vi "WorkTable Sandbox.vi"() -> ()   [LabVIEW 2011]
uses:
  Vec3d Class/Vec3d Class.lvclass
  WorkTable Class.lvclass
panel:
  out "Syringe":T1
  out "Tool Rack":T2
  in  "Config Folder":path=path "C:/Users/husker/Desktop/gantry/Config"
  out "Weights":T3
  out "Stamps":T4
  out "Manifold":T5
  out "BBM":T6
  out "Glue Reservoir":T7
  out "error out":errorcluster
  out "HDI":T8
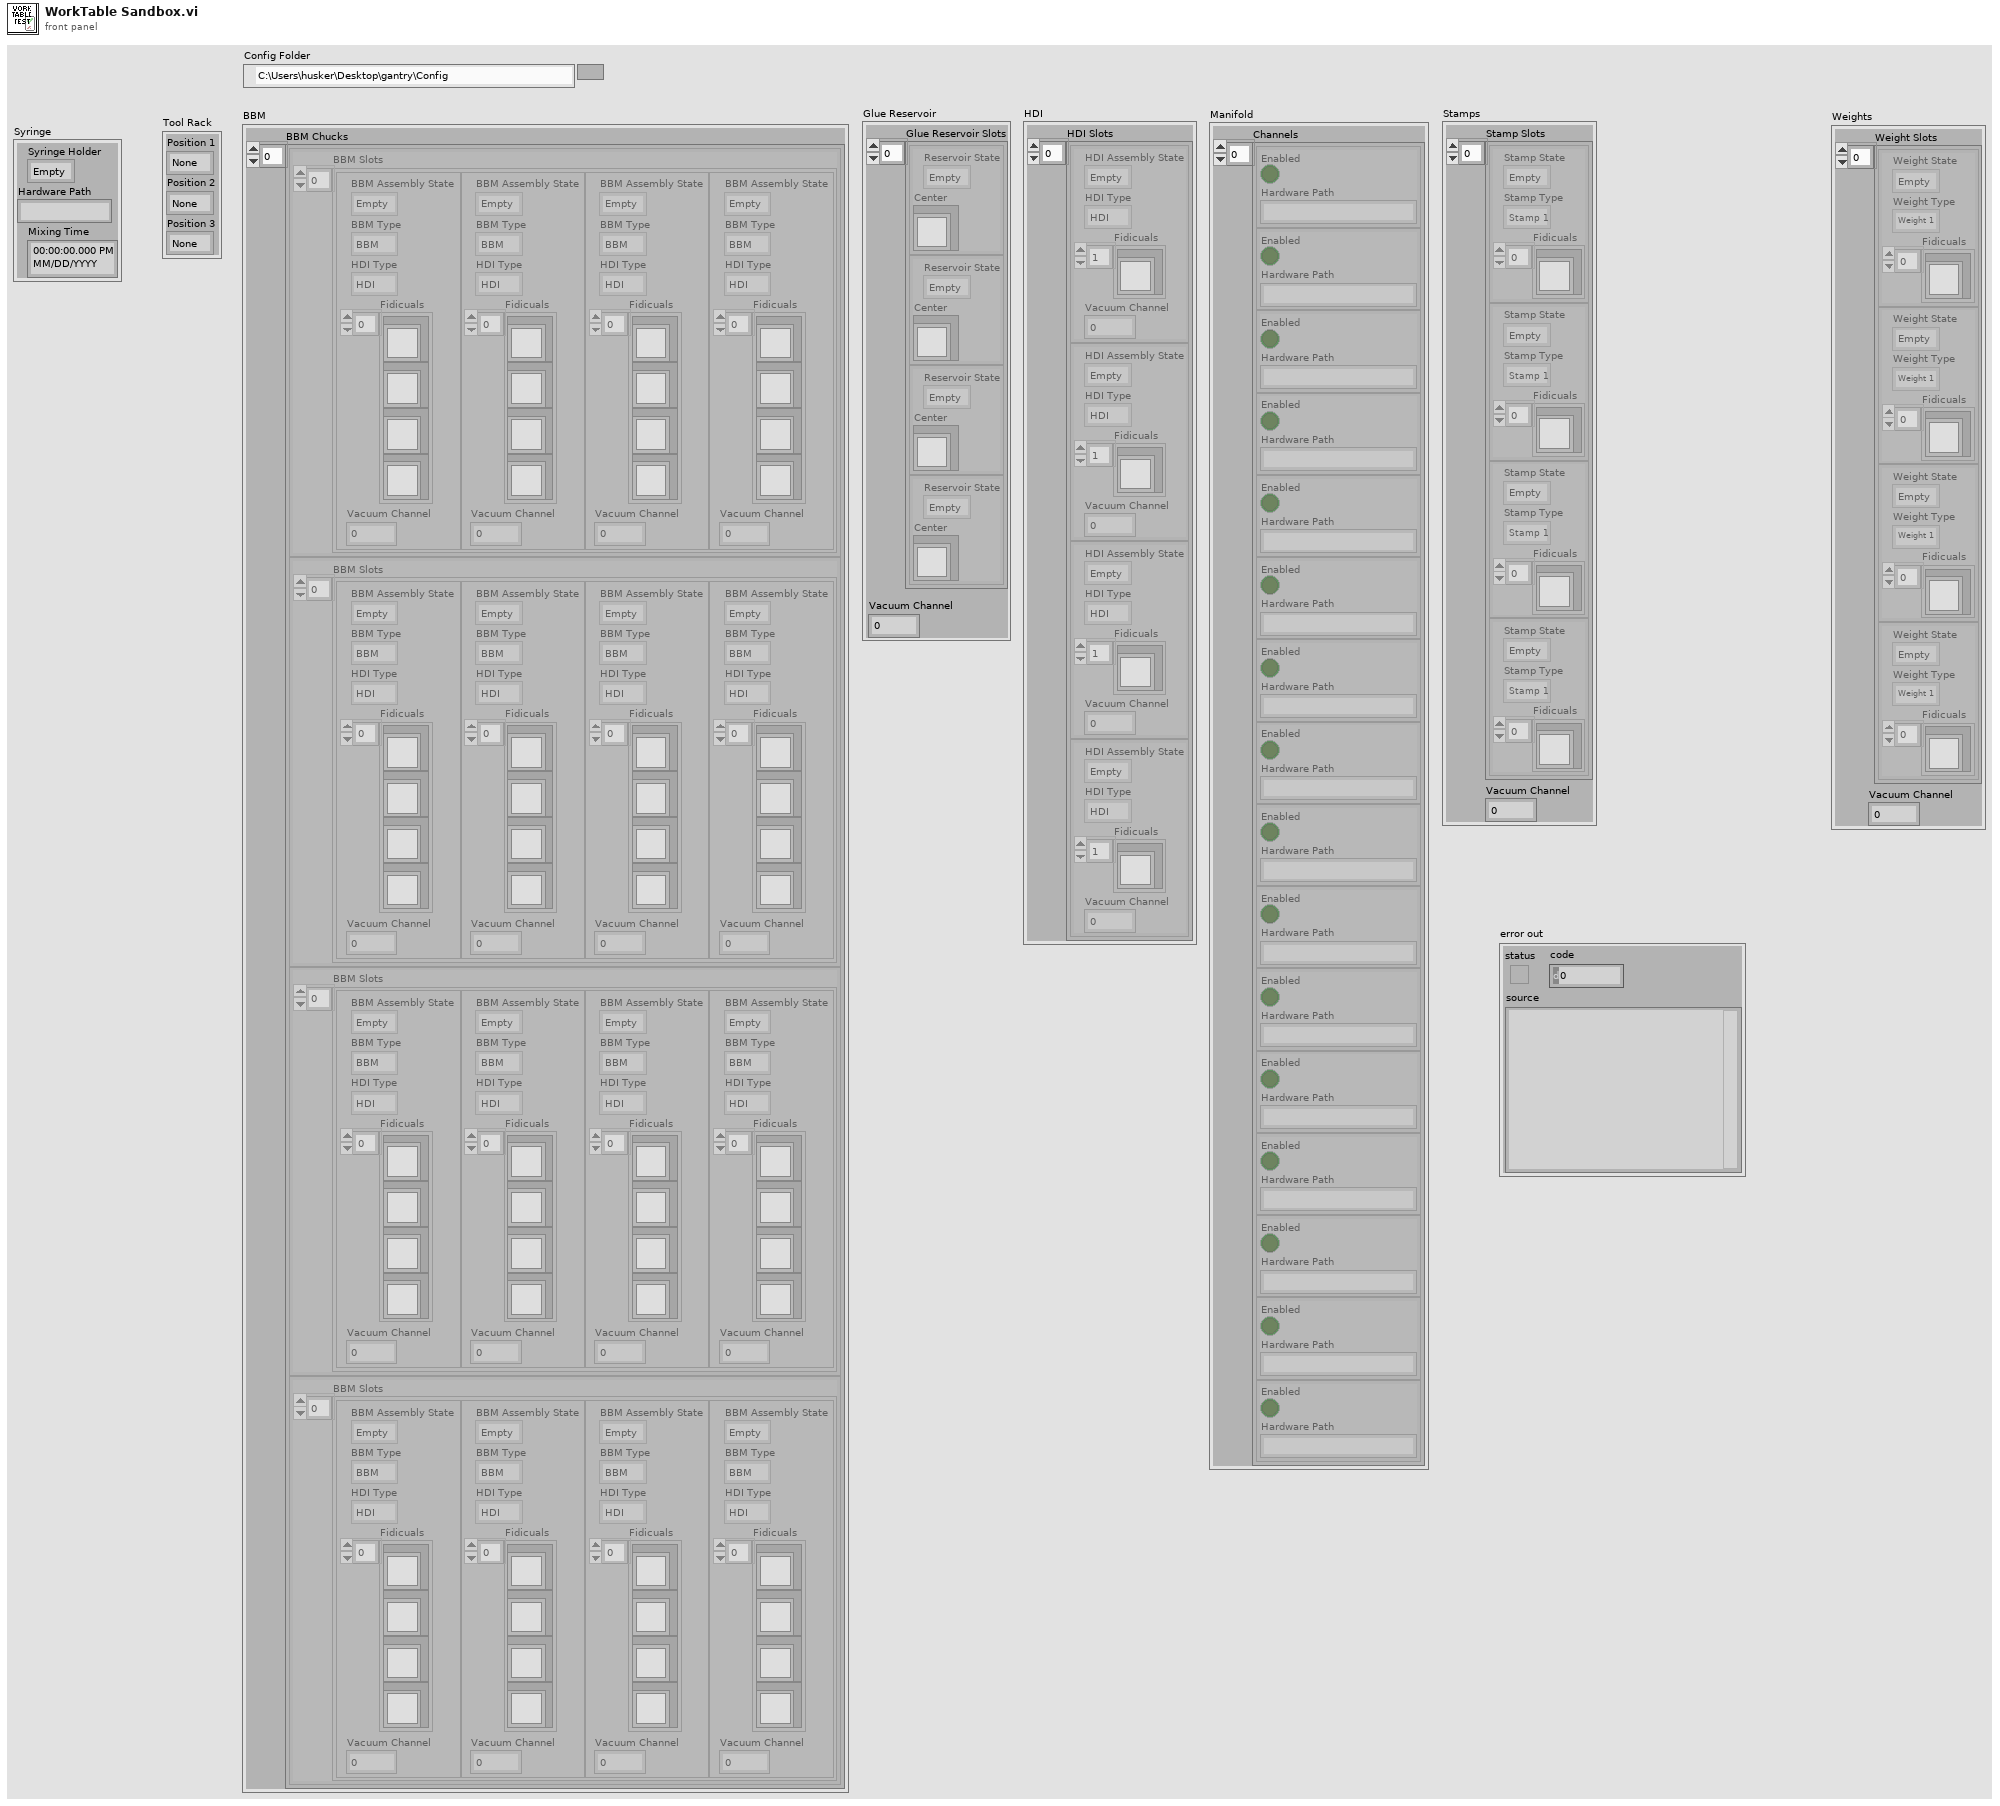
[diagram p1: front panel]
types:
  T1 = cluster{"Syringe Holder":enum16{"Empty", "Populated", "Calibrated"}, "Hardware Path":string, "Mixing Time":timestamp}
  T2 = cluster{"Position 1":enum16{"None", "Grabber", "Picker", "Tool Setter"}, "Position 2":enum16{"None", "Grabber", "Picker", "Tool Setter"}, "Position 3":enum16{"None", "Grabber", "Picker", "Tool Setter"}}
  T3 = cluster{"Weight Slots":cluster{"Weight State":enum16{"Empty", "Populated"}, "Weight Type":enum16{"Weight 1", "Weight 2", "Weight 3", "Weight 4"}, "Fidicuals":refnum<class "Vec3d Class.lvclass">[]}[], "Vacuum Channel":u8}
  T4 = cluster{"Stamp Slots":cluster{"Stamp State":enum16{"Empty", "Populated", "Used"}, "Stamp Type":enum16{"Stamp 1", "Stamp 2", "Stamp 3", "Stamp 4"}, "Fidicuals":refnum<class "Vec3d Class.lvclass">[]}[], "Vacuum Channel":u8}
  T5 = cluster{"Channels":cluster{"Enabled":bool, "Hardware Path":string}[]}
  T6 = cluster{"BBM Chucks":cluster{"BBM Slots":cluster{"BBM Assembly State":enum16{"Empty", "Unglued", "Stamped", "PartOnTop", "Weighted"}, "BBM Type":enum16{"BBM", "GlassSlide"}, "HDI Type":enum16{"HDI", "Polyimide"}, "Fidicuals":refnum<class "Vec3d Class.lvclass">[], "Vacuum Channel":u8}[]}[]}
  T7 = cluster{"Glue Reservoir Slots":cluster{"Reservoir State":enum16{"Empty", "Full", "Used"}, "Center":refnum<class "Vec3d Class.lvclass">}[], "Vacuum Channel":u8}
  T8 = cluster{"HDI Slots":cluster{"HDI Assembly State":enum16{"Empty", "Populated"}, "HDI Type":enum16{"HDI", "Polyimide"}, "Fidicuals":refnum<class "Vec3d Class.lvclass">[], "Vacuum Channel":u8}[]}
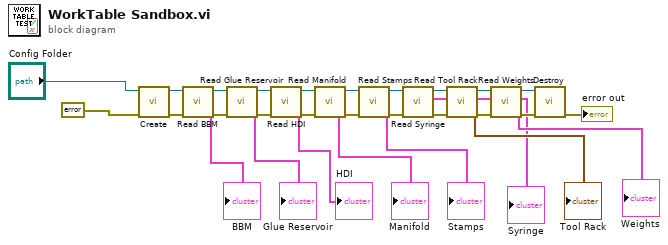
[diagram p0: block diagram]
diagram:
  n1 = call "Create.vi"("error in (no error)"=errorcluster {"status"=FALSE, "code"=0, "source"=""} ("error constant"), "Config Folder"="Config Folder") -> ("error out"=w19:errorcluster, "WorkTable Class out"=w27:refnum<class "WorkTable Class.lvclass">)  [unwired: 8 in]
  n2 = call-dynamic "Read BBM.vi"("error in (no error)"=w19, "WorkTable Class in"=w27) -> ("error out"=w18:errorcluster, "BBM"=→"BBM":T6, "WorkTable Class out"=w26:refnum<class "WorkTable Class.lvclass">)  [unwired: 7 in]
  n3 = call-dynamic "Read Glue Reservoir.vi"("error in (no error)"=w18, "WorkTable Class in"=w26) -> ("error out"=w17:errorcluster, "Glue Reservoir"=→"Glue Reservoir":T7, "WorkTable Class out"=w25:refnum<class "WorkTable Class.lvclass">)  [unwired: 7 in]
  n4 = call-dynamic "Read HDI.vi"("error in (no error)"=w17, "WorkTable Class in"=w25) -> ("error out"=w16:errorcluster, "HDI"=→"HDI":T8, "WorkTable Class out"=w24:refnum<class "WorkTable Class.lvclass">)  [unwired: 7 in]
  n5 = call-dynamic "Read Manifold.vi"("error in (no error)"=w16, "WorkTable Class in"=w24) -> ("error out"=w15:errorcluster, "Manifold"=→"Manifold":T5, "WorkTable Class out"=w23:refnum<class "WorkTable Class.lvclass">)  [unwired: 7 in]
  n6 = call-dynamic "Read Stamps.vi"("error in (no error)"=w15, "WorkTable Class in"=w23) -> ("error out"=w14:errorcluster, "Stamps"=→"Stamps":T4, "WorkTable Class out"=w22:refnum<class "WorkTable Class.lvclass">)  [unwired: 7 in]
  n7 = call-dynamic "Read Syringe.vi"("error in (no error)"=w14, "WorkTable Class in"=w22) -> ("error out"=w13:errorcluster, "Syringe"=→"Syringe":T1, "WorkTable Class out"=w21:refnum<class "WorkTable Class.lvclass">)  [unwired: 7 in]
  n8 = call-dynamic "Read Tool Rack.vi"("error in (no error)"=w13, "WorkTable Class in"=w21) -> ("error out"=w12:errorcluster, "Tool Rack"=→"Tool Rack":T2, "WorkTable Class out"=w20:refnum<class "WorkTable Class.lvclass">)  [unwired: 7 in]
  n9 = call-dynamic "Read Weights.vi"("error in (no error)"=w12, "WorkTable Class in"=w20) -> ("error out"=w11:errorcluster, "Weights"=→"Weights":T3, "WorkTable Class out"=w9:refnum<class "WorkTable Class.lvclass">)  [unwired: 7 in]
  n10 = call "Destroy.vi"("error in (no error)"=w11, "WorkTable Class.lvclass"=w9) -> ("error out"=→"error out":errorcluster)  [unwired: 9 in]
